vi "Get SMO PGSQL Log Paths.vi"(5 "getAll Cluster":variant, 7 "Paths":string="llab_038:d000(TEST_TABLE--Temperature(Kelvin))\nllab_038:d002(TEST_TABLE--voltage 2(volts))\nllab_038:b000(TEST_TABLE--ON?())\nllab_038:v001(TEST_TABLE--sample())", 8 "error in (no error)":errorcluster, 11 "Inst.TSL210 in":refnum<class "Inst.TSL210.lvclass">) -> (0 "error out":errorcluster, 2 "Paths":string, 3 "Inst.TSL210 out":refnum<class "Inst.TSL210.lvclass">)   [LabVIEW 2019, in "Inst.TSL210.lvclass"]
uses:
  Inst.TSL210.lvclass
  Typedefs/Inst.TSL210.getAll--Cluster.ctl
  <userlib>/LevyLab/Instrument Framework/Instrument Types/VSource/Instrument.VSource.lvclass
  <userlib>/LevyLab/LV-Data/LV-Data.PG/LV-Data.PGSQL.lvclass
  <userlib>/LevyLab/LV-Data/LV-Data.PG/API/Write Variable (one-row).vi
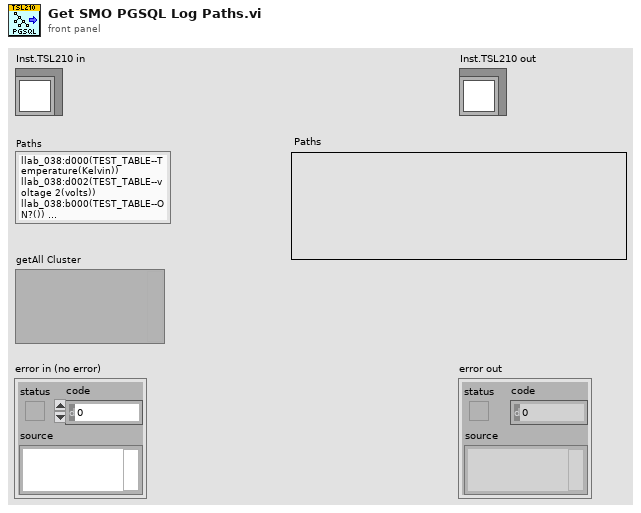
[diagram p1: front panel]
types:
  T1 = typedef "Inst.TSL210.lvclass/Inst.TSL210.getAll--Cluster.ctl" = cluster{"Wavelength (nm)":dbl, "Power (mW)":dbl, "Status: LD":bool, "Status: COH":bool, "Status: TempError":bool, "Status: CurrentLimit":bool, "Status: SystemBusy":bool, "Status: ATT":bool, "Status: ACC":bool, "Status: FT":bool}
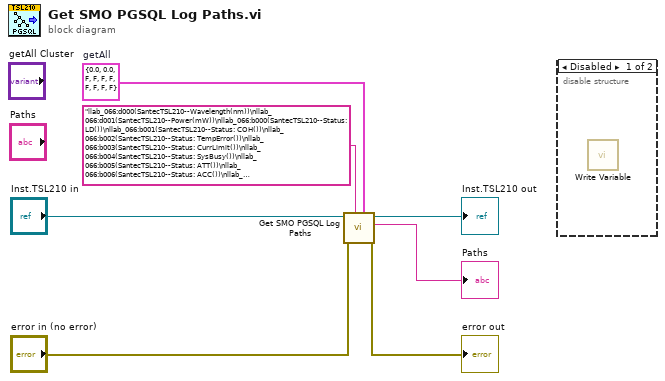
[diagram p0: block diagram]
diagram:
  w1 = T1 {"Wavelength (nm)"=0.0, "Power (mW)"=0.0, "Status: LD"=FALSE, "Status: COH"=FALSE, "Status: TempError"=FALSE, "Status: CurrentLimit"=FALSE, "Status: SystemBusy"=FALSE, "Status: ATT"=FALSE, "Status: ACC"=FALSE, "Status: FT"=FALSE}  # getAll
  n1 = call-parent "Get SMO PGSQL Log Paths.vi"("getAll Cluster"=w1, "Default Paths"="llab_066:d000(SantecTSL210--Wavelength(nm))\nllab_066:d001(SantecTSL210--Power(mW))\nllab_066:b000(SantecTSL210--Status: LD())\nllab_066:b001(SantecTSL210--Status: COH())\nllab_066:b002(SantecTSL210--Status: TempError())\nllab_066:b003(SantecTSL210--Status: CurrLimit())\nllab_066:b004(SantecTSL210--Status: SysBusy())\nllab_066:b005(SantecTSL210--Status: ATT())\nllab_066:b006(SantecTSL210--Status: ACC())\nllab_066:b007(SantecTSL210--Status: FT())" ("Paths"), "error in (no error)"="error in (no error)", "Instrument in"="Inst.TSL210 in") -> ("error out"=→"error out":errorcluster, "Paths"=→"Paths":string, "Instrument out"=→"Inst.TSL210 out":refnum<class "Inst.TSL210.lvclass">)  [unwired: 5 in]
  n2 = disable-structure shown="Disabled" {
    frame Disabled {
      n3 = call-poly <userlib>:"Write Variable.vi"() -> ()  [unwired: 8 in, 4 out]
    }
    frame Enabled {
    }
  }
